vi "Calculadora - Cristhian Tipan.vi"() -> ()   [LabVIEW 2020]
panel:
  in  "stop":bool
  in  "FUNCIONES":T1(ring)
  out "RESULTADO":dbl
  in  "NUM 2":dbl
  in  "NUM 1":dbl
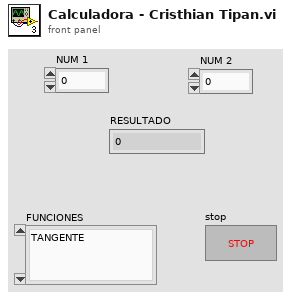
[diagram p1: front panel]
types:
  T1 = enum16{"TANGENTE", "COSENO", "SENO", "EXPONENCIAL", "CONVERSION GRADOS A RADIANES", "RAIZ CUADRADA", "DIVISION", "MULTIPLICACION", "RESTA", "SUMA"}
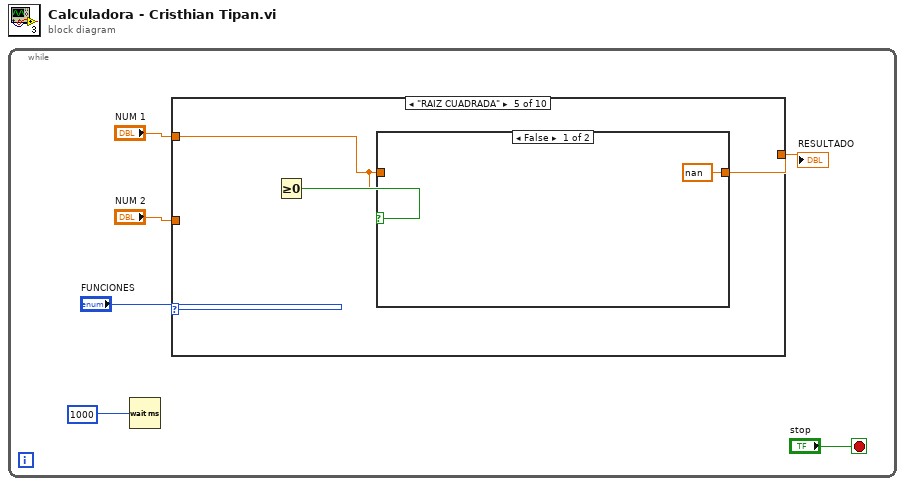
[diagram p0: block diagram]
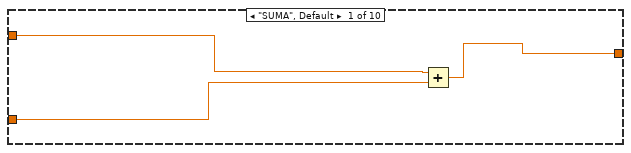
[diagram p2: hidden frame]
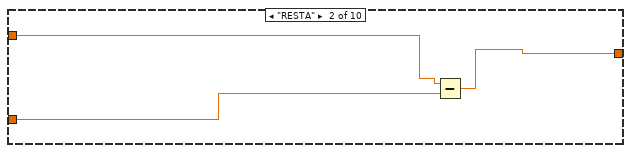
[diagram p3: hidden frame]
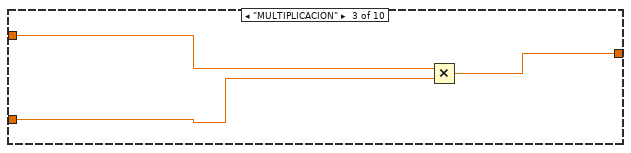
[diagram p4: hidden frame]
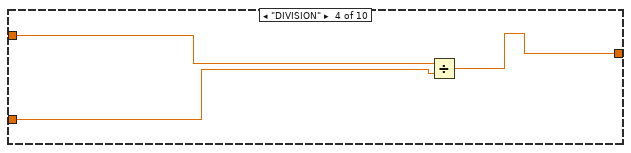
[diagram p5: hidden frame]
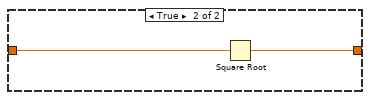
[diagram p6: hidden frame]
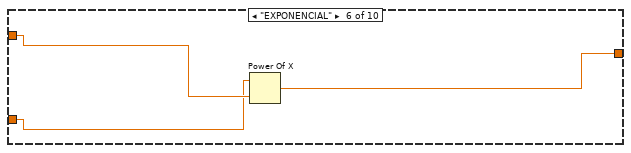
[diagram p7: hidden frame]
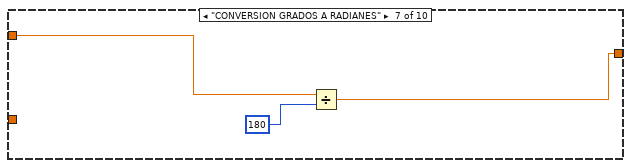
[diagram p8: hidden frame]
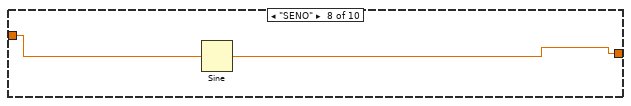
[diagram p9: hidden frame]
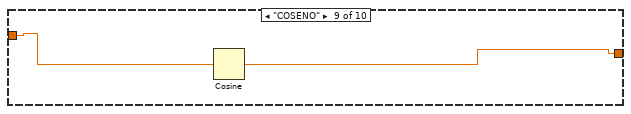
[diagram p10: hidden frame]
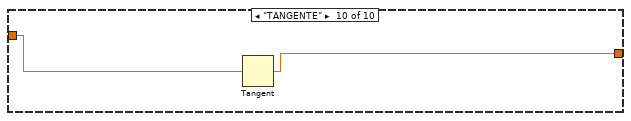
[diagram p11: hidden frame]
diagram:
  n1 = while {
    stop <- "stop" stop-if-true
    n2 = Wait (ms)(milliseconds to wait=1000) -> ()  [unwired: 1 out]
    n3 = case shown="\"RAIZ CUADRADA\"" "FUNCIONES" {
      tunnel: "NUM 1" -> [w9 w12 w15 w18 w19 w26 w28 w32 w34 w36]
      tunnel: "NUM 2" -> [w8 w11 w14 w17 _ w25 _ _ _ _]
      tunnel: [w7 w10 w13 w16 w20 w27 w29 w31 w33 w35] -> w4
      frame "SUMA", Default {
        n4 = Add(x=w9, y=w8) -> (x+y=w7:dbl)
      }
      frame "RESTA" {
        n5 = Subtract(x=w12, y=w11) -> (x-y=w10:dbl)
      }
      frame "MULTIPLICACION" {
        n6 = Multiply(x=w15, y=w14) -> (x*y=w13:dbl)
      }
      frame "DIVISION" {
        n7 = Divide(x=w18, y=w17) -> (x/y=w16:dbl)
      }
      frame "RAIZ CUADRADA" {
        n8 = Greater Or Equal To 0?(x=w19) -> (x >= 0?=w21:bool)
        n9 = case shown="False" w21 {
          tunnel: [nan w24] -> w20
          tunnel: w19 -> [_ w23]
          frame False {
          }
          frame True {
            n10 = Square Root(x=w23) -> (sqrt(x)=w24:dbl)
          }
        }
      }
      frame "EXPONENCIAL" {
        n11 = Power Of X(1:w26, 2:w25) -> (0:w27:dbl)
      }
      frame "CONVERSION GRADOS A RADIANES" {
        n12 = Divide(x=w28, y=180) -> (x/y=w29:dbl)
      }
      frame "SENO" {
        n13 = Sine(x=w32) -> (sin(x)=w31:dbl)
      }
      frame "COSENO" {
        n14 = Cosine(x=w34) -> (cos(x)=w33:dbl)
      }
      frame "TANGENTE" {
        n15 = Tangent(1:w36) -> (0:w35:dbl)
      }
    }
    "RESULTADO" <- w4
  }
